vi "Find Nested LV XML.vi"(8 "error in (no error)":errorcluster, 11 "Projext Path":path) -> (0 "error out":errorcluster, 2 "lvlibs":path[](array[path]), 3 "lvprojs":path[](array[path]))   [LabVIEW 2020, in "Test Finder.lvclass"]
uses:
  Test Finder.lvclass
  Test Finder.lvclass/Test Finder.ctl
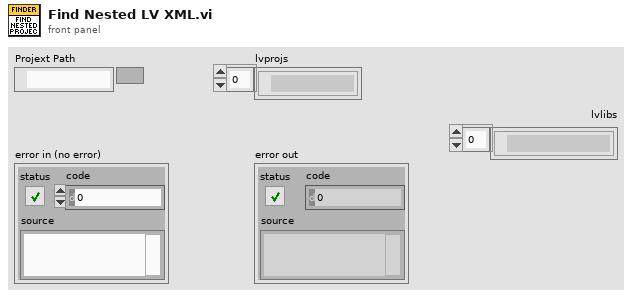
[diagram p1: front panel]
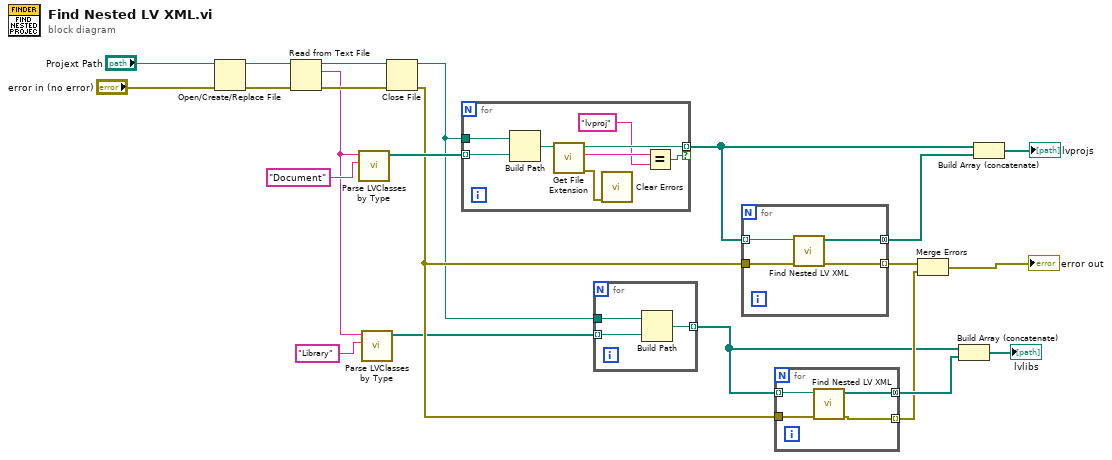
[diagram p0: block diagram]
diagram:
  n1 = Open/Create/Replace File(file path (use dialog)="Projext Path", error in="error in (no error)") -> (refnum out=w17:refnum<file>, error out=w18:errorcluster)  [unwired: 4 in, 1 out]
  n2 = Read from Text File(file (use dialog)=w17, error in=w18) -> (refnum out=w19:refnum<file>, text=w8:string, error out=w20:errorcluster)  [unwired: 2 in, 1 out]
  n3 = call "Parse LVClasses by Type.vi"("Type"="Document", "Input"=w8) -> ("Relative Paths"=w15:path[])  [unwired: 9 in]
  n4 = call "Parse LVClasses by Type.vi"("Type"="Library", "Input"=w8) -> ("Relative Paths"=w2:path[])  [unwired: 9 in]
  n5 = Close File(refnum=w19, error in=w20) -> (path=w3:path, error out=w5:errorcluster)
  n6 = for {
    tunnel: w3 -> [w30]
    tunnel: w15 -> [w29] mode=indexing
    tunnel: [w27] -> w14 mode=indexing if=w23
    n7 = Build Path(base path=w30, name or relative path=w29) -> (appended path=w28:path)
    n8 = call <vilib>:"Get File Extension.vi"("file"=w28) -> ("error out"=w24:errorcluster, "lowercase file extension"=w26:string, "dup file"=w27:path)  [unwired: 6 in, 2 out]
    n9 = call <vilib>:"Clear Errors.vi"("error in (no error)"=w24) -> ()  [unwired: 5 in, 2 out]
    n10 = Equal?(x=w26, y="lvproj") -> (x = y?=w23:bool)
  }
  n11 = for {
    tunnel: w3 -> [w33]
    tunnel: w2 -> [w32] mode=indexing
    tunnel: [w31] -> w1 mode=indexing
    n12 = Build Path(base path=w33, name or relative path=w32) -> (appended path=w31:path)
  }
  n13 = for {
    tunnel: w14 -> [w37] mode=indexing
    tunnel: [w36] -> w12 mode=concatenating
    tunnel: w5 -> [w35]
    tunnel: [w34] -> w11 mode=indexing
    n14 = call "Find Nested LV XML.vi"("error in (no error)"=w35, "Projext Path"=w37) -> ("error out"=w34:errorcluster, "lvprojs"=w36:path[])  [unwired: 7 in, 1 out]
  }
  n15 = for {
    tunnel: w1 -> [w41] mode=indexing
    tunnel: [w40] -> w6 mode=concatenating
    tunnel: w5 -> [w39]
    tunnel: [w38] -> w4 mode=indexing
    n16 = call "Find Nested LV XML.vi"("error in (no error)"=w39, "Projext Path"=w41) -> ("error out"=w38:errorcluster, "lvprojs"=w40:path[])  [unwired: 7 in, 1 out]
  }
  n17 = Merge Errors(w11, w4) -> (→"error out":errorcluster)
  n18 = Build Array (concatenate)(w1, w6) -> (→"lvlibs":path[])
  n19 = Build Array (concatenate)(w14, w12) -> (→"lvprojs":path[])
